vi "OSN_Query.vi"(0 "System no.":i32=1 min=1 max=4 step=1, 2 "Channel to query":string[](array[string]), 3 "All channels?":bool, 4 "Channel identifier?":bool=TRUE, 5 "error in":errorcluster) -> (14 "No. of steps left":i32[](array[numeric]), 19 "error out":errorcluster)   [LabVIEW 2020]
doc: "Returns the number of steps still to be performed for the given channel or axis after the last OSM command.\n\nC-891: If All channels = TRUE, then Axis identifier can be FALSE.\n\nE-712: If All channels = TRUE, then Axis identifier must be FALSE. \n\nE-755: If All channels = TRUE, then Axis identifier must be FALSE\n\nE-872: If All channels = TRUE, then Axis identifier must be FALSE.\n\nE-871, E-873: If All channels = TRUE, then Axis identifier must be FALSE. \nE-135, E-874: If All channels = TRUE, then Axis identifier must be FALSE."
panel:
  # "Returns the number of steps left from the number of steps set by\nlast OSM command for the given Nexline channel."
  # "If all channels: use"
  # "Query"
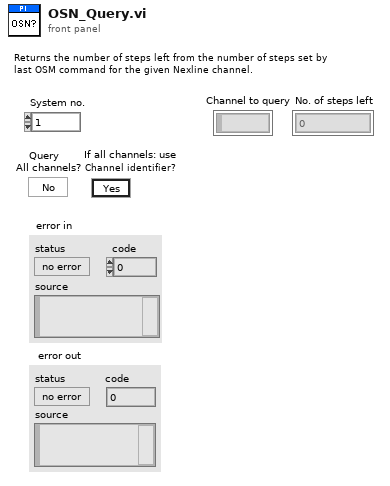
[diagram p1: front panel]
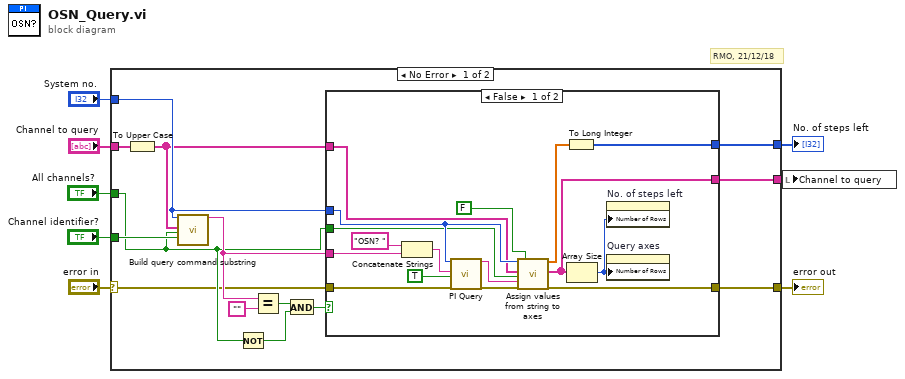
[diagram p0: block diagram]
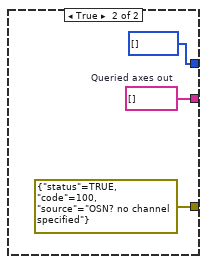
[diagram p2: hidden frame]
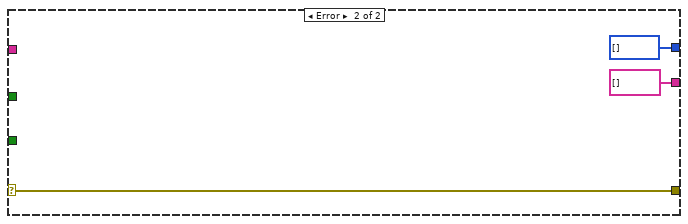
[diagram p3: hidden frame]
diagram:
  # "RMO, 21/12/18"
  n1 = case shown="No Error" "error in" {
    selector: "error in" -> [w9 w42]
    tunnel: [w22 i32[] []] -> w8
    tunnel: "Channel to query" -> [w21 _]
    tunnel: [w11 w42] -> w6
    tunnel: "Channel identifier?" -> [w19 _]
    tunnel: "System no." -> [w17 _]
    tunnel: [w13 string[] [] ("Axes to query out")] -> w3
    tunnel: "All channels?" -> [w16 _]
    frame No Error {
      n2 = To Upper Case(1:w21) -> (0:w12:string[])
      n3 = call "Build query command substring.vi"("System no."=w17, "Axes to query in"=w12, "Query\nAll axes?"=w16, "For all axes: use\nAxis identifier?"=w19) -> ("Command substring"=w18:string)  [unwired: 2 in, 13 out]
      n4 = Not(x=w16) -> (.not. x?=w14:bool)
      n5 = Equal?(x=w18, y="" ("x")) -> (x = y?=w15:bool)
      n6 = And(x=w15, y=w14) -> (x .and. y?=w10:bool)
      n7 = case shown="False" w10 {
        tunnel: [w23 i32[] []] -> w22
        tunnel: w18 -> [w35 _]
        tunnel: w17 -> [w34 _]
        tunnel: w16 -> [w33 _]
        tunnel: [w31 w39] -> w13
        tunnel: w12 -> [w29 _]
        tunnel: [w28 errorcluster {"status"=TRUE, "code"=100, "source"="OSN? no channel specified"} ("error out")] -> w11
        tunnel: w9 -> [w25 _]
        frame False {
          n8 = Concatenate Strings("OSN? ", w35) -> (w36:string)
          n9 = call "PI Query.vi"("System no."=w34, "String to send"=w36, "Attach termination char.?"=TRUE ("Attach Linefeed?"), "error in"=w25) -> ("String read"=w26:string, "error out"=w27:errorcluster)  [unwired: 3 in, 11 out]
          n10 = call "Assign values from string to axes.vi"("System no."=w34, "Queried axes"=w29, "All axes queried?"=w33, "Input String"=w26, "error in"=w27, "Axes related?"=FALSE) -> ("Values"=w24:dbl[], "Queried axes out"=w31:string[], "error out"=w28:errorcluster)  [unwired: 3 in, 8 out]
          n11 = To Long Integer(number=w24) -> (32bit integer=w23:i32[])
          n12 = Array Size(array=w31) -> (size(s)=w30:i32)
          n13 = property on="No. of steps left" class="Arr (strict)"("Number of Rows"=w30) -> ()  [unwired: 2 in, 2 out]
          n14 = property on="Query axes" class="Arr (strict)"("Number of Rows"=w30) -> ()  [unwired: 2 in, 2 out]
        }
        frame True {
          w39 = string[] []  # Queried axes out
        }
      }
    }
    frame Error {
    }
  }
  "error out" <- w6
  "No. of steps left" <- w8
  n15 = local write "Channel to query"(w3) -> ()
